vi "Gradient descent ideal diode.vi"() -> ()   [LabVIEW 2011]
panel:
  out "DelV-t":cluster{i32[], dbl[]}(graph)
  in  "Learning rate":dbl
  out "First Gradient in loop":dbl
  out "First V in loop":dbl
  out "P-t":cluster{dbl[], dbl[]}(graph)
  out "P-V":cluster{dbl[], dbl[]}(graph)
  out "J-V":cluster{dbl[], dbl[]}(graph)
  out "Vmp-t":cluster{dbl[], dbl[]}(graph)
  in  "MaxPow Stabilisation time (s)":dbl
  in  "Initial voltage":dbl
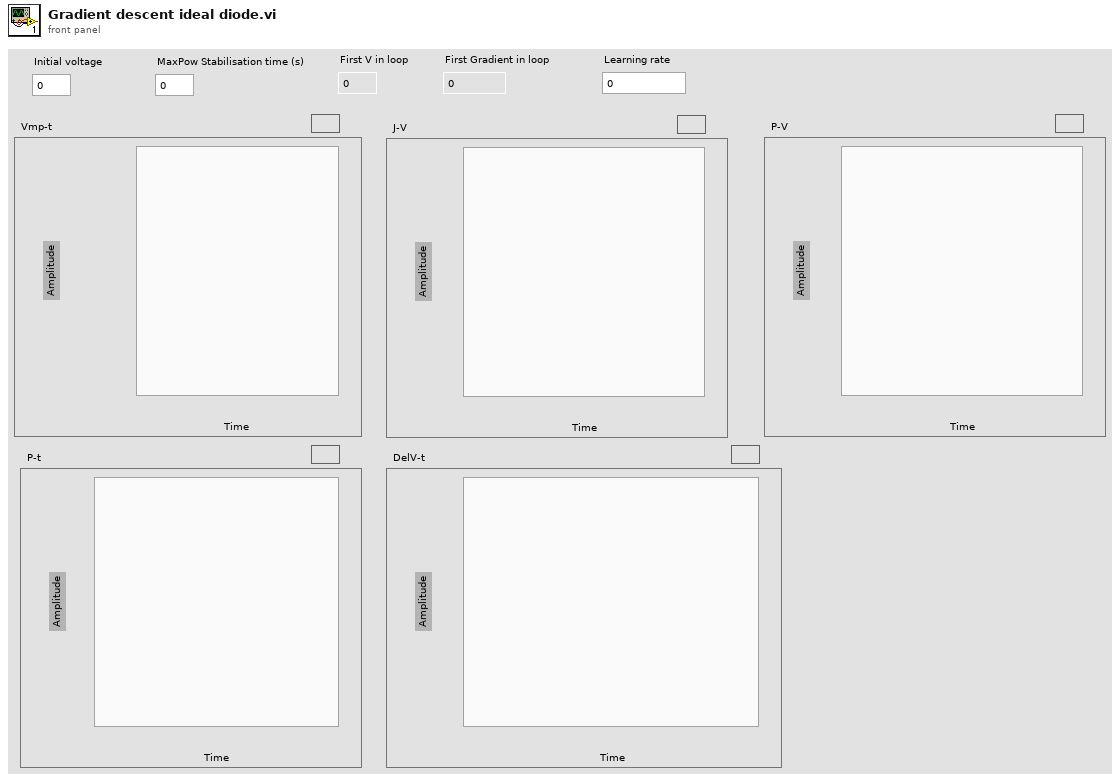
[diagram p1: front panel]
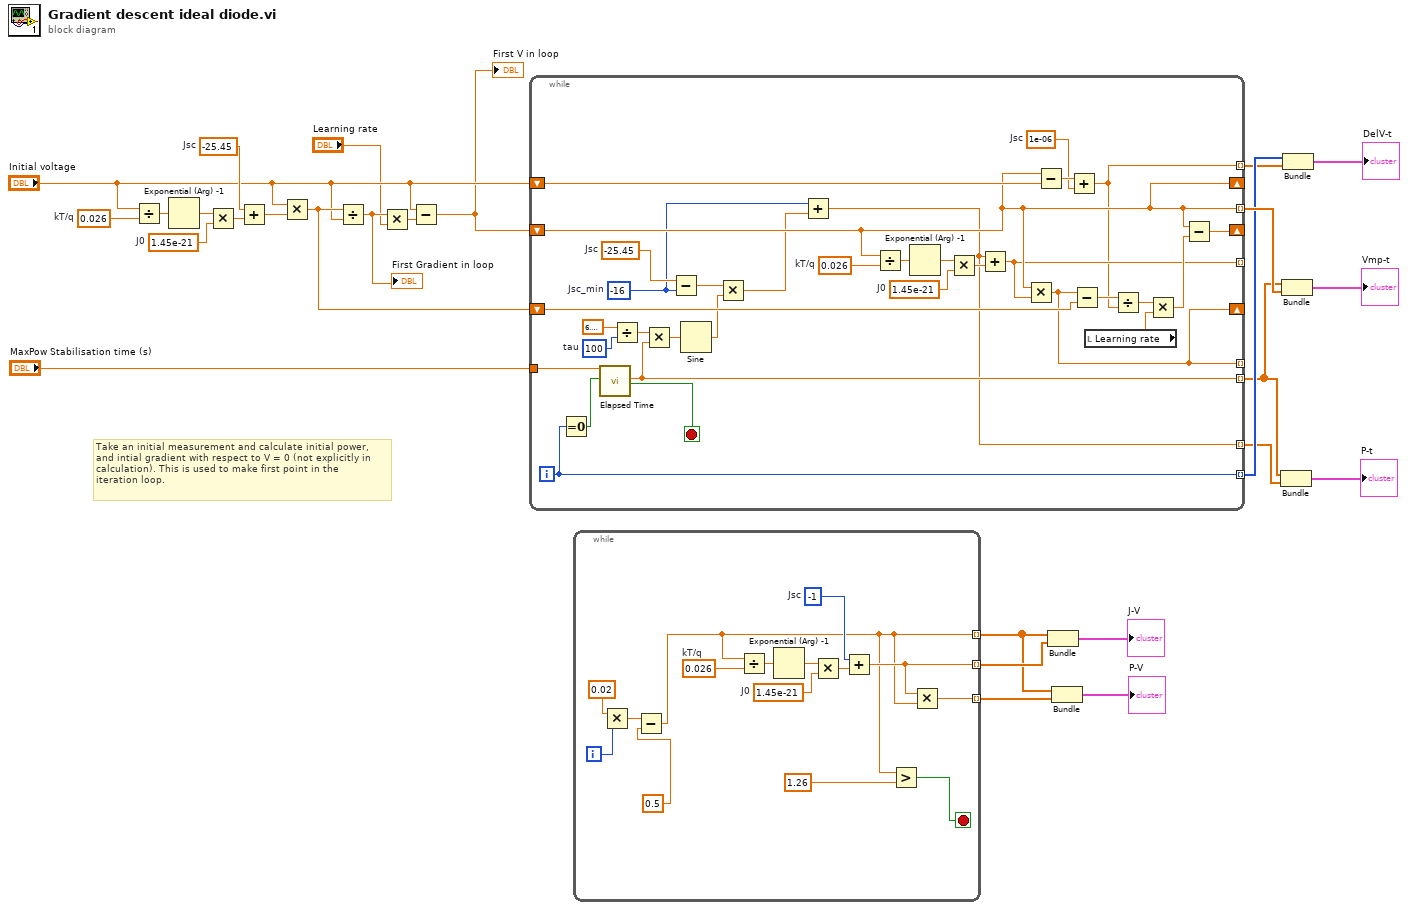
[diagram p0: block diagram]
diagram:
  w24 = 0.026  # kT/q
  w19 = -25.45  # Jsc
  w21 = 1.45e-21  # J0
  # "Take an initial measurement and calculate initial power,\nand intial gradient with respect to V = 0 (not explicitly in\ncalculation). This is used to make first point in the\niteration loop."
  n1 = Divide(x="Initial voltage", y=w24) -> (x/y=w23:dbl)
  n2 = Exponential (Arg) -1(1:w23) -> (0:w22:dbl)
  n3 = Multiply(x=w22, y=w21) -> (x*y=w20:dbl)
  n4 = Add(x=w19, y=w20) -> (x+y=w18:dbl)
  n5 = Multiply(x="Initial voltage", y=w18) -> (x*y=w25:dbl)
  n6 = Divide(x=w25, y="Initial voltage") -> (x/y=w7:dbl)
  "First Gradient in loop" <- w7
  n7 = Multiply(x=w7, y="Learning rate") -> (x*y=w27:dbl)
  n8 = Subtract(x="Initial voltage", y=w27) -> (x-y=w9:dbl)
  "First V in loop" <- w9
  n9 = while {
    tunnel: [w38] -> w1 mode=indexing
    tunnel: [w44] -> _ mode=indexing
    tunnel: "MaxPow Stabilisation time (s)" -> [w58]
    shift-right: [w52] -> _
    shift-left: w9 -> [w45]
    shift-right: [w51] -> _
    shift-left: w25 -> [w57]
    shift-right: [w45] -> _
    shift-left: "Initial voltage" -> [w55]
    tunnel: [w51] -> _ mode=indexing
    tunnel: [w45] -> w16 mode=indexing
    tunnel: [w43] -> w4 mode=indexing
    tunnel: [w29] -> w3 mode=indexing
    tunnel: [w33] -> w2 mode=indexing
    i -> [w43]
    stop <- w60 stop-if-true
    w28 = 1e-06  # Jsc
    w31 = -16  # Jsc_min
    w40 = 100  # tau
    w35 = -25.45  # Jsc
    w46 = 0.026  # kT/q
    w49 = 1.45e-21  # J0
    n10 = Equal To 0?(x=w43) -> (x = 0?=w59:bool)
    n11 = call "Elapsed Time"("Time Target (s)"=w58, "Reset"=w59) -> ("Elapsed Time (s)"=w38:dbl, "Time has Elapsed"=w60:bool)  [unwired: 10 in, 6 out]
    n12 = Divide(x=6.283185307179586, y=w40) -> (x/y=w39:dbl)
    n13 = Multiply(x=w39, y=w38) -> (x*y=w37:dbl)
    n14 = Subtract(x=w35, y=w31) -> (x-y=w32:dbl)
    n15 = Sine(x=w37) -> (sin(x)=w36:dbl)
    n16 = Multiply(x=w32, y=w36) -> (x*y=w34:dbl)
    n17 = Add(x=w31, y=w34) -> (x+y=w33:dbl)
    n18 = Divide(x=w45, y=w46) -> (x/y=w47:dbl)
    n19 = Exponential (Arg) -1(1:w47) -> (0:w48:dbl)
    n20 = Multiply(x=w48, y=w49) -> (x*y=w50:dbl)
    n21 = Add(x=w33, y=w50) -> (x+y=w44:dbl)
    n22 = Multiply(x=w45, y=w44) -> (x*y=w51:dbl)
    n23 = Subtract(x=w45, y=w55) -> (x-y=w30:dbl)
    n24 = Add(x=w30, y=w28) -> (x+y=w29:dbl)
    n25 = Subtract(x=w51, y=w57) -> (x-y=w56:dbl)
    n26 = local read "Learning rate"() -> (w42:dbl)
    n27 = Divide(x=w56, y=w29) -> (x/y=w54:dbl)
    n28 = Multiply(x=w54, y=w42) -> (x*y=w53:dbl)
    n29 = Subtract(x=w45, y=w53) -> (x-y=w52:dbl)
  }
  n30 = while {
    tunnel: [w61] -> w11 mode=indexing
    tunnel: [w65] -> w13 mode=indexing
    tunnel: [w64] -> w10 mode=indexing
    i -> [w69]
    stop <- w66 stop-if-true
    w75 = 0.026  # kT/q
    w70 = -1  # Jsc
    w72 = 1.45e-21  # J0
    n31 = Multiply(x=0.02, y=w69) -> (x*y=w63:dbl)
    n32 = Subtract(x=w63, y=0.5) -> (x-y=w61:dbl)
    n33 = Divide(x=w61, y=w75) -> (x/y=w74:dbl)
    n34 = Exponential (Arg) -1(1:w74) -> (0:w73:dbl)
    n35 = Multiply(x=w73, y=w72) -> (x*y=w71:dbl)
    n36 = Add(x=w70, y=w71) -> (x+y=w65:dbl)
    n37 = Greater?(x=w61, y=1.26) -> (0:w66:bool)
    n38 = Multiply(x=w65, y=w61) -> (x*y=w64:dbl)
  }
  n39 = Bundle(w11, w13) -> (→"J-V":cluster{dbl[], dbl[]})  [unwired: 1 in]
  n40 = Bundle(w11, w10) -> (→"P-V":cluster{dbl[], dbl[]})  [unwired: 1 in]
  n41 = Bundle(w1, w2) -> (→"P-t":cluster{dbl[], dbl[]})  [unwired: 1 in]
  n42 = Bundle(w1, w16) -> (→"Vmp-t":cluster{dbl[], dbl[]})  [unwired: 1 in]
  n43 = Bundle(w4, w3) -> (→"DelV-t":cluster{i32[], dbl[]})  [unwired: 1 in]
